vi "Cooler State Trace.vi"(4 "error in (no error)":errorcluster, 6 "Launch Order":i32, 7 "Cooler State":enum16{"Off", "On"}(ring)) -> (0 "error out":errorcluster)   [LabVIEW 2020, in "Startup Processes.lvlib"]
uses:
  Startup Processes.lvlib
  toolbox/Debugging/Debugging.lvlib
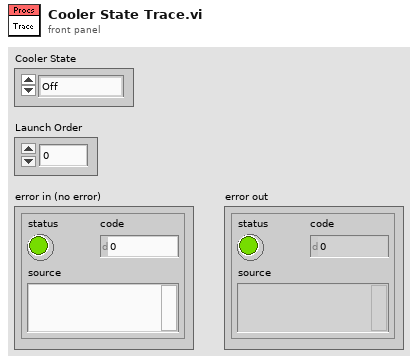
[diagram p1: front panel]
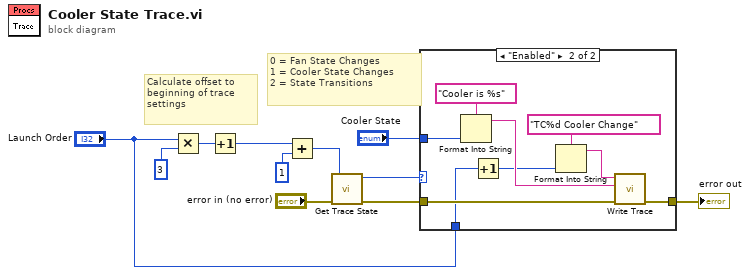
[diagram p0: block diagram]
diagram:
  # "0 = Fan State Changes\n1 = Cooler State Changes\n2 = State Transitions"
  # "Calculate offset to beginning of trace settings"
  n1 = Multiply(x="Launch Order", y=3) -> (x*y=w10:i32)
  n2 = Increment(x=w10) -> (x+1=w9:i32)
  n3 = Add(x=w9, y=1) -> (x+y=w3:i32)
  n4 = call "Get Trace State.vi"("Error In"="error in (no error)", "Trace Point Index"=w3) -> ("Error Out"=w7:errorcluster, "Trace Point State"=w6:enum16{"Disabled", "Enabled"})  [unwired: 4 in]
  n5 = case shown="\"Enabled\"" w6 {
    tunnel: w7 -> [w12 w21]
    tunnel: [w12 w20] -> w4
    tunnel: "Cooler State" -> [_ w19]
    tunnel: "Launch Order" -> [_ w13]
    frame "Disabled" {
    }
    frame "Enabled" {
      n6 = Format Into String(format string="Cooler is %s", w19) -> (resulting string=w18:string)  [unwired: 2 in, 1 out]
      n7 = Increment(x=w13) -> (x+1=w15:i32)
      n8 = Format Into String(format string="TC%d Cooler Change" ("Trace Point Name"), w15) -> (resulting string=w16:string)  [unwired: 2 in, 1 out]
      n9 = call "Write Trace.vi"("Error In"=w21, "Trace Data"=w18, "Trace Point Name"=w16) -> ("Error Out"=w20:errorcluster)  [unwired: 4 in]
    }
  }
  "error out" <- w4
